vi "Open.vi"(8 "error in":errorcluster, 9 "Timeout":i32=-1 format="%.0f ms", 11 "Reply Protocol in":refnum<class "Reply Protocol Base.lvclass">) -> (0 "error out":errorcluster, 3 "Reply Protocol out":refnum<class "Reply Protocol Base.lvclass">)   [LabVIEW 2023, in "HAL GOOP4.lvlib" / "Reply Protocol Base.lvclass"]
uses:
  Reply Protocol Base.lvclass
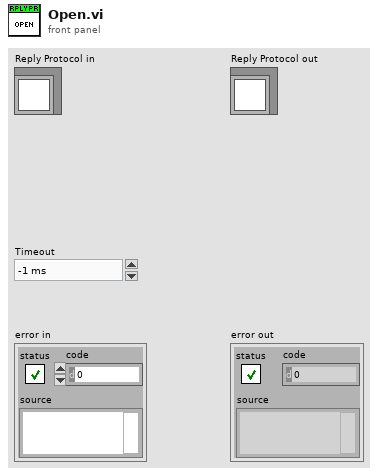
[diagram p1: front panel]
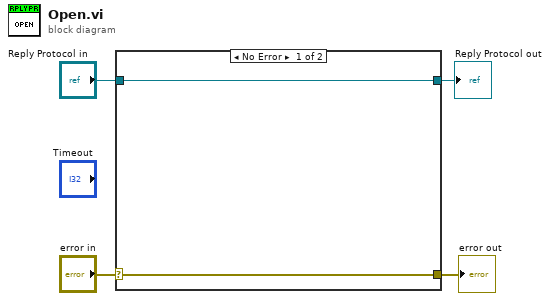
[diagram p0: block diagram]
diagram:
  n1 = case shown="No Error" "error in" {
    selector: "error in" -> [w6 w8]
    tunnel: [w6 w8] -> w3
    tunnel: "Reply Protocol in" -> [w5 w7]
    tunnel: [w5 w7] -> w1
    frame No Error {
    }
    frame Error {
    }
  }
  "error out" <- w3
  "Reply Protocol out" <- w1
